vi "GetMap.vi"(0 "object in":refnum<class "Map.lvclass">, 5 "error in (no error)":errorcluster) -> (14 "object out":refnum<class "Map.lvclass">, 16 "Grid":u32[][](array[colorbox]), 19 "error out":errorcluster)   [LabVIEW 2015, in "Map.lvclass"]
doc: "Returns the map grid."
uses:
  Map.lvclass
  Map.lvclass/Map.ctl
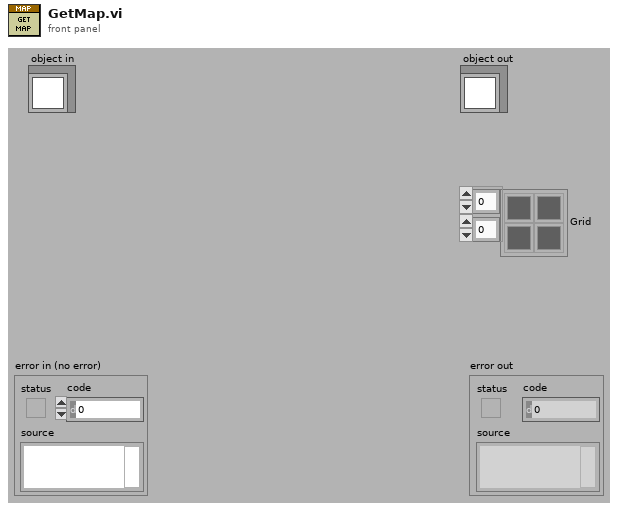
[diagram p1: front panel]
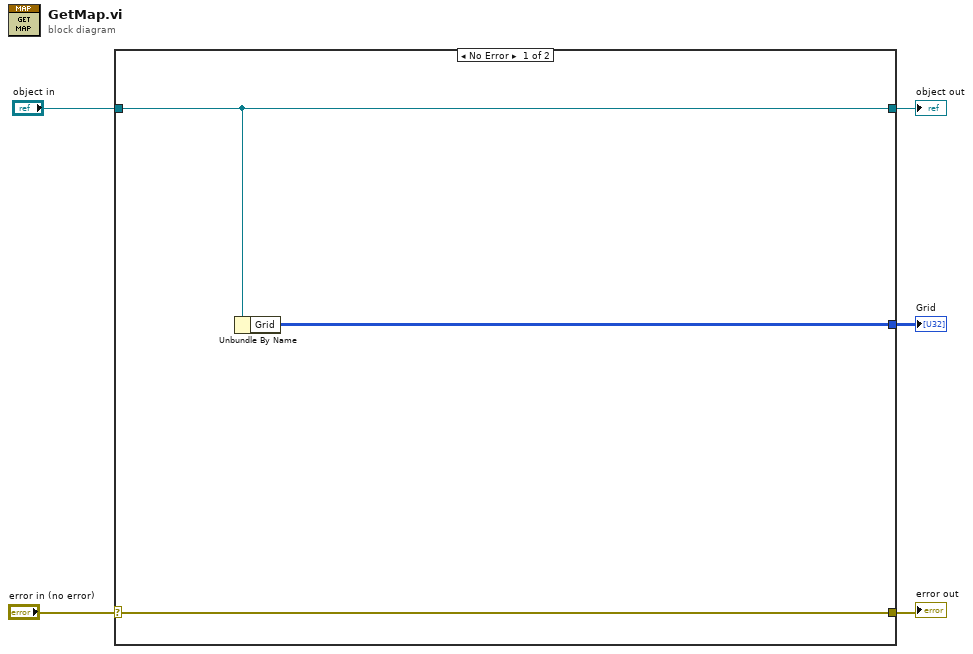
[diagram p0: block diagram]
diagram:
  n1 = case shown="No Error" "error in (no error)" {
    selector: "error in (no error)" -> [w7 w10]
    tunnel: [w7 w10] -> w4
    tunnel: [w8 w9] -> w2
    tunnel: "object in" -> [w8 w9]
    tunnel: [w6 _] -> w1
    frame No Error {
      n2 = Unbundle By Name(w8) -> ("Grid"=w6:u32[][])
    }
    frame Error {
    }
  }
  "error out" <- w4
  "object out" <- w2
  "Grid" <- w1
